vi "Process Functional Array.vi"(11 "Function Array":T1[](array[typedef])) -> (2 "Complete Array":bool, 3 "Number Array":i32[](array[numeric]))   [LabVIEW 2023]
uses:
  ENUM_Type.ctl
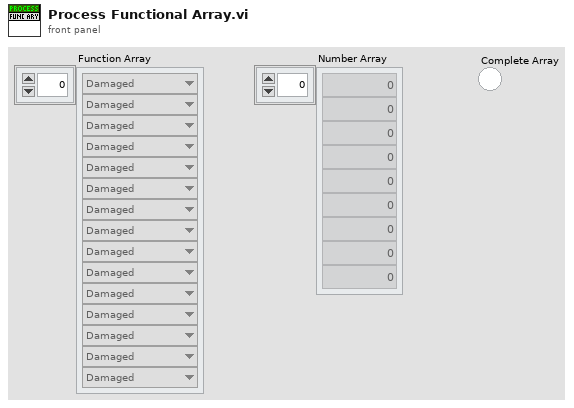
[diagram p1: front panel]
types:
  T1 = typedef "ENUM_Type.ctl" = enum16{"Damaged", "Operational", "Unknown"}
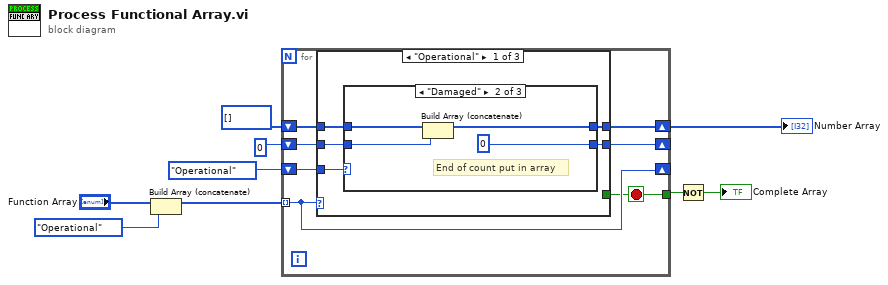
[diagram p0: block diagram]
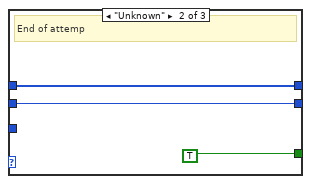
[diagram p4: hidden frame]
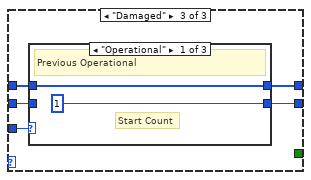
[diagram p5: hidden frame]
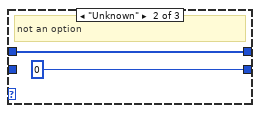
[diagram p6: hidden frame]
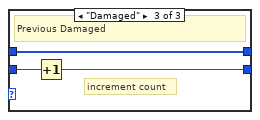
[diagram p7: hidden frame]
diagram:
  n1 = Build Array (concatenate)("Function Array", ENUM_Type."Operational" ("Enum")) -> (w2:T1[])
  n2 = for {
    tunnel: w2 -> [w11] mode=indexing
    shift-right: [w11] -> _
    shift-left: ENUM_Type."Operational" ("Enum") -> [w16]
    shift-right: [w12] -> w7
    shift-left: i32[] [] ("Number Array") -> [w15]
    shift-right: [w13] -> _
    shift-left: 0 ("String") -> [w14]
    tunnel: [w10] -> w8
    stop <- w10 stop-if-true
    n3 = case shown="\"Operational\"" w11 {
      tunnel: w16 -> [w21 _ w37]
      tunnel: w15 -> [w19 w32 w36]
      tunnel: w14 -> [w20 w31 w35]
      tunnel: [w17 w31 w34] -> w13
      tunnel: [w18 w32 w33] -> w12
      tunnel: [_ TRUE _] -> w10
      frame "Operational" {
        n4 = case shown="\"Damaged\"" w21 {
          tunnel: w20 -> [w22 w26 w28]
          tunnel: w19 -> [w23 w27 w29]
          tunnel: [w23 w25 w29] -> w18
          tunnel: [w22 0 ("String") w28] -> w17
          frame "Operational" {
            # "Do nothing"
          }
          frame "Damaged" {
            # "End of count put in array"
            n5 = Build Array (concatenate)(w27, w26) -> (w25:i32[])
          }
          frame "Unknown" {
          }
        }
      }
      frame "Unknown" {
        # "End of attemp"
      }
      frame "Damaged" {
        n6 = case shown="\"Operational\"" w37 {
          tunnel: w36 -> [w38 w40 w42]
          tunnel: w35 -> [_ _ w44]
          tunnel: [1 0 w43] -> w34
          tunnel: [w38 w40 w42] -> w33
          frame "Operational" {
            # "Start Count"
            # "Previous Operational"
          }
          frame "Unknown" {
            # "not an option"
          }
          frame "Damaged" {
            # "increment count"
            # "Previous Damaged"
            n7 = Increment(x=w44) -> (x+1=w43:i32)
          }
        }
      }
    }
  }
  "Number Array" <- w7
  n8 = Not(x=w8) -> (.not. x?=→"Complete Array":bool)
